vi "cyclone Special Features.vi"(4 "paramReference2":u32, 5 "paramReference1":u32, 6 "paramValue3":u32, 7 "paramValue2":u32, 9 "paramValue1":u32, 10 "setFeature":bool, 11 "featureNum":u32) -> (1 "function return":bool, 2 "paramReference2 out":u32, 3 "paramReference1 out":u32)   [LabVIEW 2021, in "CycloneControlSDK.lvlib"]
doc: "extern \"C\" bool _cdecl cycloneSpecialFeatures(uint32_t featureNum, bool setFeature, uint32_t paramValue1, uint32_t paramValue2, uint32_t paramValue3, void *paramReference1, void *paramReference2);"
uses:
  CycloneControlSDK.lvlib
  CycloneControlSDK_64.dll
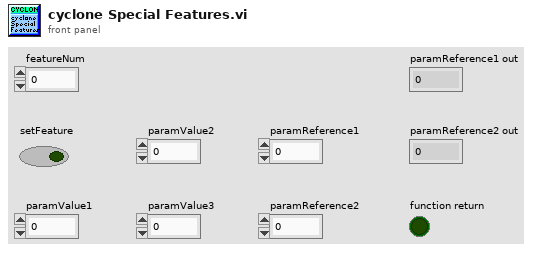
[diagram p1: front panel]
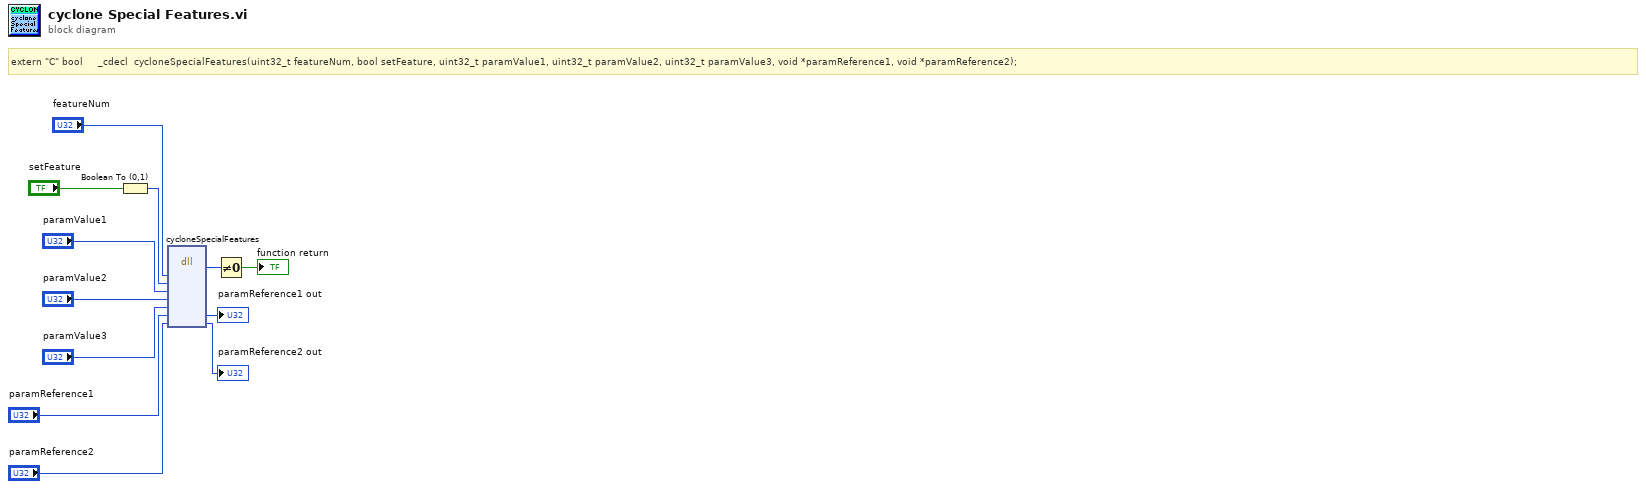
[diagram p0: block diagram]
diagram:
  # "extern \"C\" bool     _cdecl  cycloneSpecialFeatures(uint32_t featureNum, bool setFeature, uint32_t paramValue1, uint32_t paramValue2, uint32_t paramValue3, void *paramReference1, void *paramReference2);"
  n1 = Boolean To (0,1)(Boolean="setFeature") -> (0, 1=w8:i16)
  n2 = dll-call lib="C:/PEMicro/cyclone/cycloneControl/controlsdk/examples/labview2018/user.lib/CycloneControlSDK/CycloneControlSDK_64.dll" fn="cycloneSpecialFeatures"("featureNum"="featureNum", "setFeature"=w8, "paramValue1"="paramValue1", "paramValue2"="paramValue2", "paramValue3"="paramValue3", "paramReference1"="paramReference1", "paramReference2"="paramReference2") -> ("return type"=w11:u8, "paramReference1"=→"paramReference1 out":u32, "paramReference2"=→"paramReference2 out":u32)  [unwired: 8 in, 2 out]
  n3 = Not Equal To 0?(x=w11) -> (x != 0?=→"function return":bool)
